vi "Modbus_Stop_FVIR_Test.vi"(8 "error in (no error)":errorcluster, 11 "Queue in":refnum<queue>) -> (0 "error out":errorcluster)   [LabVIEW 2020]
uses:
  support/Message Queue/Message Cluster.ctl
  support/Message Queue/Enqueue Message (Single).vi
  support/Message Queue/Message Queue.lvlib
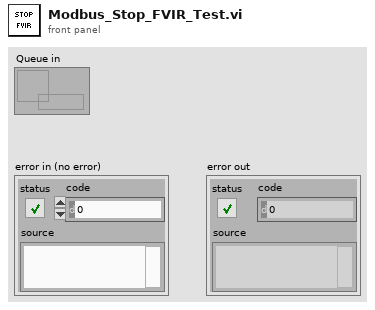
[diagram p1: front panel]
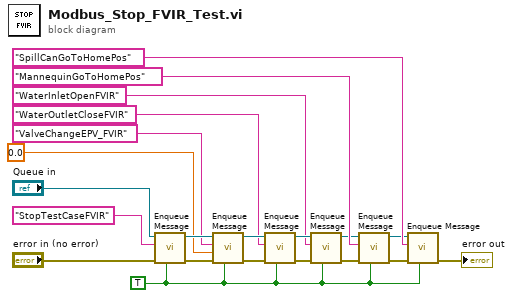
[diagram p0: block diagram]
diagram:
  w1 = TRUE ("Priority Message? (F)")
  n1 = call-poly "Enqueue Message.vi"("Priority Message? (F)"=w1, "error in (no error)"="error in (no error)", "Message"="StopTestCaseFVIR", "Message Queue"="Queue in") -> ("error out"=w10:errorcluster, "dup Message Queue"=w9:refnum<queue>)  [unwired: 6 in]
  n2 = call-poly "Enqueue Message.vi"("Priority Message? (F)"=w1, "error in (no error)"=w10, "Message Data"=0.0 ("Proportioning Valve 2"), "Message"="ValveChangeEPV_FVIR", "Message Queue"=w9) -> ("error out"=w12:errorcluster, "dup Message Queue"=w13:refnum<queue>)  [unwired: 5 in]
  n3 = call-poly "Enqueue Message.vi"("Priority Message? (F)"=w1, "error in (no error)"=w12, "Message"="WaterOutletCloseFVIR", "Message Queue"=w13) -> ("error out"=w15:errorcluster, "dup Message Queue"=w16:refnum<queue>)  [unwired: 6 in]
  n4 = call-poly "Enqueue Message.vi"("Priority Message? (F)"=w1, "error in (no error)"=w15, "Message"="WaterInletOpenFVIR", "Message Queue"=w16) -> ("error out"=w21:errorcluster, "dup Message Queue"=w3:refnum<queue>)  [unwired: 6 in]
  n5 = call-poly "Enqueue Message.vi"("Priority Message? (F)"=w1, "error in (no error)"=w21, "Message"="MannequinGoToHomePos", "Message Queue"=w3) -> ("error out"=w18:errorcluster, "dup Message Queue"=w17:refnum<queue>)  [unwired: 6 in]
  n6 = call-poly "Enqueue Message.vi"("Priority Message? (F)"=w1, "error in (no error)"=w18, "Message"="SpillCanGoToHomePos", "Message Queue"=w17) -> ("error out"=→"error out":errorcluster)  [unwired: 6 in, 1 out]
